vi "Configure Level Trigger.vi"(0 "device session in":refnum<class "Device Session.lvclass">, 1 "trigger source":u8, 5 "trigger when":T1, 7 "trigger level (V)":dbl, 11 "error in":errorcluster, 12 "instance":enum16{"A", "B"}(ring)) -> (4 "device session out":refnum<class "Device Session.lvclass">, 15 "error out":errorcluster)   [LabVIEW 2021, in "Device Session.lvclass"]
doc: "Configures the level trigger for a channel. You can specify the trigger slope, the trigger level, and whether the device should trigger on an input below or above the specified trigger level. You must run the <B>Configure Channel</B> VI before running this VI.\n\n<B>Input Parameters</B>\n\n<B>device session in</B> is a reference to the Device Session object, which contains a session to each instrument design library used in this sample project. This parameter is obtained from the 'Open Session' VI.\n\n<B>trigger source</B> specifies the channel to monitor for trigger conditions.\n\n<B>trigger when</B> specifies whether the device should trigger if the input is below or above the specified 'level'.\n\n<B>trigger level (V)</B> specifies the voltage threshold for the trigger.\n\n<B>instance</B> specifies either instance A or B of the trigger to use.\n\n<B>error in</B> describes error conditions that occur before this node runs. This input provides standard 'error in' functionality.\n\n<B>Output Parameters</B>\n\n<B>device session out</B> passes a reference to the session to the next VI.\n\n<B>error out</B> contains error information. This output provides standard 'error out' functionality."
uses:
  Device Session.lvclass
  FPGA Refnum.ctl
  <vilib>/rvi/interface/nirviReadWriteControl/nirviReadWriteControl.xnode
  <vilib>/rvi/interface/Simulation/niFpgaSimulationCallBeginRW.vi
  <vilib>/rvi/errors/niLvFpgaAdjustHostInterfaceError.vi
  <instrlib>/_niInstr/Data Trigger/v1/Shared/Public/Level Configuration Trigger When.ctl
  <instrlib>/_niInstr/Data Trigger/v1/Shared/niInstr Data Trigger v1 Shared.lvlib
  <instrlib>/_niInstr/Data Trigger/v1/Shared/Public/Level Configuration FXP(+-,18,1).ctl
  NiFpgaLv.dll
  <vilib>/Utility/error.llb/Error Cluster From Error Code.vi
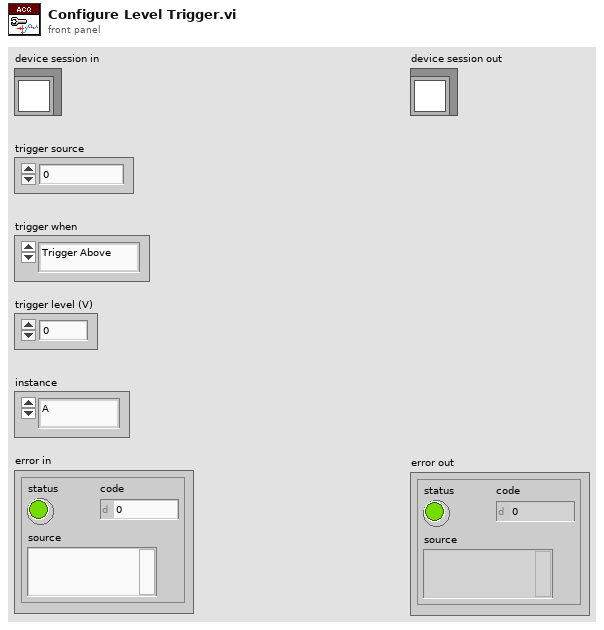
[diagram p1: front panel]
types:
  T1 = typedef "niInstr Data Trigger v1 Shared.lvlib/Level Configuration Trigger When.ctl" = enum8{"Trigger Above", "Trigger Below"}
  T2 = typedef "niInstr Data Trigger v1 Shared.lvlib/Level Configuration FXP(+-,18,1).ctl" = cluster{"level":fxp<+/-,18,1>, "trigger when":T1}
  T3 = enum16{"Immediate", "A", "B", "OR", "AND", "A THEN B", "B THEN A", "High Resolution"}
  T4 = typedef "Device Session.lvclass/Device Session Object.ctl" = cluster{"fpga reference":T5, "reg bus":refnum<class "niInstr FIFO Register Bus v1 Host.lvclass">, "subsystem map":refnum<class "niInstr Subsystem Map v1 Host.lvclass">, "cal data":refnum<class "niHSAI Cal Data v1 Host.lvclass">, "config":refnum<class "niHSAI Group A Config v1 Host.lvclass">, "acquisition":refnum<class "niInstr Multirecord Acquisition v1 Host.lvclass">, "number of selected acq channels":u8, "selected acq channels":bool[], "number of channels":u32, "configured channels":bool[], "acq configuration":cluster{"number of samples":u64, "number of records":u64, "pretrigger samples":u64}, "actual channel configuration":T6[], "sample clock rate (Hz)":dbl, "scaling coefficients":T10[]}
  T5 = typedef "Device Session.lvclass/FPGA Refnum.ctl" = refnum<k20>
  T6 = typedef "niHSAI Types v1 Host.lvlib/Channel Configuration.ctl" = cluster{"channel":u32, "coupling":T7, "impedance":T8, "bandwidth":T9, "vertical range":dbl, "vertical offset":dbl}
  T7 = typedef "niHSAI Types v1 Host.lvlib/Coupling.ctl" = enum8{"Default", "DC", "AC"}
  T8 = typedef "niHSAI Types v1 Host.lvlib/Impedance.ctl" = enum8{"Default", "1 mega ohm", "50 ohm"}
  T9 = typedef "niHSAI Types v1 Host.lvlib/Bandwidth.ctl" = enum8{"Default", "Full Bandwidth", "Anti-alias Filter", "150 MHz"}
  T10 = typedef "niInstr Multirecord Acquisition v1 Host.lvclass/Scaling Coefficient.ctl" = cluster{"gain":dbl, "offset":dbl}
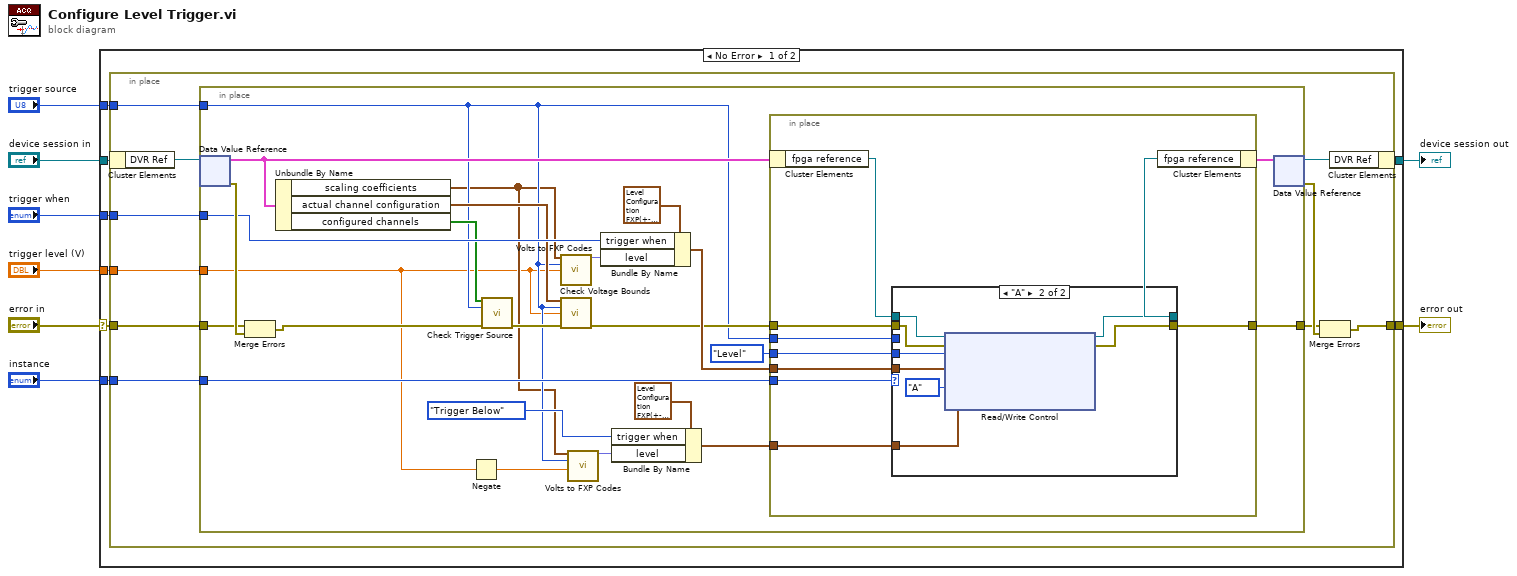
[diagram p0: block diagram]
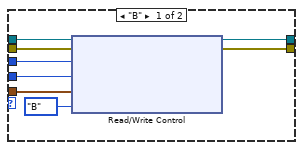
[diagram p2: hidden frame]
diagram:
  n1 = case shown="No Error" "error in" {
    selector: "error in" -> [w16 w77]
    tunnel: "device session in" -> [w10 w76]
    tunnel: [w9 w76] -> w7
    tunnel: [w11 w77] -> w8
    tunnel: "trigger source" -> [w15 _]
    tunnel: "trigger when" -> [w14 _]
    tunnel: "instance" -> [w13 _]
    tunnel: "trigger level (V)" -> [w12 _]
    frame No Error {
      n2 = in-place {
        in-place-border: w16 -> [w26]
        in-place-border: w15 -> [w25]
        in-place-border: w14 -> [w23]
        in-place-border: w13 -> [w22]
        in-place-border: w12 -> [w20]
        in-place-border: [w19] -> w11
        n3 = in-place-cluster #1(w10) -> ("DVR Ref"=w18:refnum<data-value>)
        n4 = in-place {
          in-place-border: w26 -> [w49]
          in-place-border: w25 -> [w31]
          in-place-border: w23 -> [w44]
          in-place-border: w22 -> [w47]
          in-place-border: [w46] -> w21
          in-place-border: w20 -> [w29]
          n5 = in-place-dvr #2(w18) -> (w38:T4, w50:errorcluster)
          n6 = Merge Errors(w49, w50) -> (w36:errorcluster)
          n7 = Unbundle By Name(w38) -> ("scaling coefficients"=w30:T10[], "actual channel configuration"=w35:T6[], "configured channels"=w41:bool[])
          n8 = Negate(x=w29) -> (-x=w28:dbl)
          n9 = call "Check Trigger Source.vi"("configured channels"=w41, "trigger source"=w31, "error in"=w36) -> ("error out"=w40:errorcluster)  [unwired: 12 in]
          n10 = call "Volts to FXP Codes.vi"("scaling coefficients"=w30, "channel index"=w31, "level (V)"=w29) -> ("codes"=w42:fxp<+/-,18,1>)  [unwired: 12 in]
          n11 = call "Check Voltage Bounds.vi"("channel configuration"=w35, "trigger source"=w31, "level (V)"=w29, "error in"=w40) -> ("error out"=w39:errorcluster)  [unwired: 11 in]
          n12 = call "Volts to FXP Codes.vi"("scaling coefficients"=w30, "channel index"=w31, "level (V)"=w28) -> ("codes"=w32:fxp<+/-,18,1>)  [unwired: 12 in]
          n13 = Bundle By Name(cluster=T2 {"level"=0.0, "trigger when"=enum."Trigger Above"} ("configuration"), "trigger when"=w44, "level"=w42) -> (w45:T2)
          n14 = Bundle By Name(cluster=T2 {"level"=0.0, "trigger when"=enum."Trigger Above"} ("configuration"), "trigger when"=Level_Configuration_Trigger_When."Trigger Below", "level"=w32) -> (w27:T2)
          n15 = in-place {
            in-place-border: enum16{"Edge", "Level", "Custom"}."Level" ("trigger.select 0") -> [w59]
            in-place-border: w47 -> [w58]
            in-place-border: [w57] -> w46
            in-place-border: w45 -> [w56]
            in-place-border: w39 -> [w55]
            in-place-border: w31 -> [w54]
            in-place-border: w27 -> [w51]
            n16 = in-place-cluster #3(w38) -> ("fpga reference"=w52:T5)
            n17 = case shown="\"A\"" w58 {
              tunnel: w55 -> [w67 w75]
              tunnel: w54 -> [w62 _]
              tunnel: [w66 w74] -> w53
              tunnel: [w65 w73] -> w57
              tunnel: w59 -> [w63 w72]
              tunnel: w56 -> [w64 w71]
              tunnel: w52 -> [w60 w69]
              tunnel: w51 -> [_ w68]
              frame "B" {
                n18 = xnode "Read/Write Control"("FPGA VI Reference In"=w60, "error in"=w67, "trigger.channel B"=w62, "trigger.type B"=w63, "trigger.level B"=w64, "trigger.combination type"=T3."B" ("trigger.combination.type")) -> ("FPGA VI Reference Out"=w66:T5, "error out"=w65:errorcluster)
              }
              frame "A" {
                n19 = xnode "Read/Write Control"("FPGA VI Reference In"=w69, "error in"=w75, "trigger.type A"=w72, "trigger.level A"=w71, "trigger.combination type"=T3."A" ("trigger.combination.type"), "trigger.level B"=w68) -> ("FPGA VI Reference Out"=w74:T5, "error out"=w73:errorcluster)
              }
            }
            n20 = in-place-cluster #3("fpga reference"=w53) -> (w37:T4)
          }
          n21 = in-place-dvr #2(w37) -> (w17:refnum<data-value>, w24:errorcluster)
        }
        n22 = Merge Errors(w21, w24) -> (w19:errorcluster)
        n23 = in-place-cluster #1("DVR Ref"=w17) -> (w9:refnum<class "Device Session.lvclass">)
      }
    }
    frame Error {
    }
  }
  "error out" <- w8
  "device session out" <- w7
